vi "computeSetpoints.vi"(8 "idealSPFraction":dbl=0.7 format="%#_13g", 9 "Mdot":dbl, 10 "OffIdeal":dbl, 11 "MFCsIn":T1[](array[typedef]) {"mDot" format="%_4g"; "Setpoint" format="%.2g"; "MFCcapability"."MaxMdot" format="%_4g"; "MFCcapability"."MinMdot" format="%_4g"}) -> (1 "InactiveMFCs 2":T1[](array[typedef]) {"mDot" format="%_4g"; "Setpoint" format="%.2g"; "MFCcapability"."MaxMdot" format="%_4g"; "MFCcapability"."MinMdot" format="%_4g"}, 3 "ActiveMFCs":T1[](array[typedef]) {"mDot" format="%_4g"; "Setpoint" format="%.2g"; "MFCcapability"."MaxMdot" format="%_4g"; "MFCcapability"."MinMdot" format="%_4g"})   [LabVIEW 2021]
uses:
  MFCdescription.ctl
  MFCcapability.ctl
panel:
  out "mDotTotal":dbl
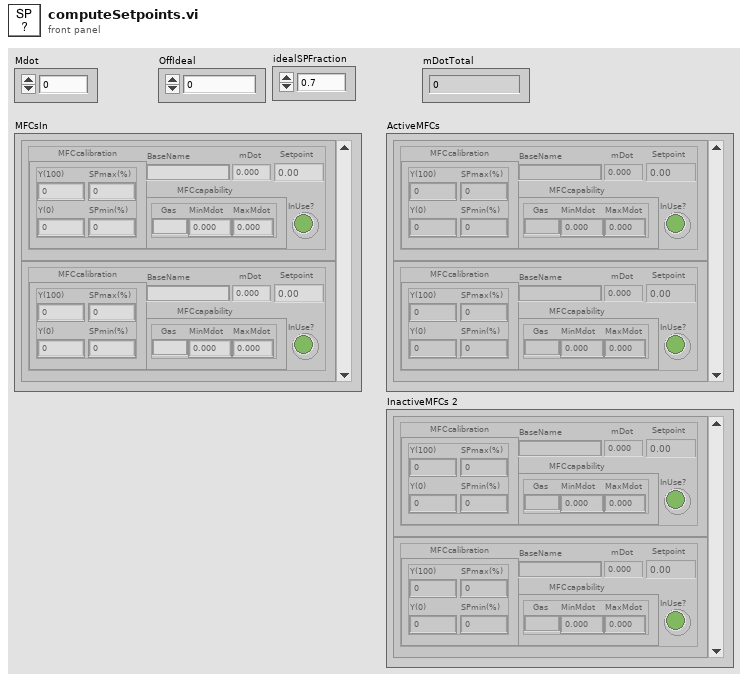
[diagram p1: front panel]
types:
  T1 = typedef "MFCdescription.ctl" = cluster{"BaseName":string, "MFCcalibration":cluster{"Y(100)":dbl, "Y(0)":dbl, "SPmin(%)":dbl, "SPmax(%)":dbl}, "MFCcapability":T2, "InUse?":bool, "Setpoint":dbl, "mDot":dbl}
  T2 = typedef "MFCcapability.ctl" = cluster{"Gas":string, "MinMdot":dbl, "MaxMdot":dbl}
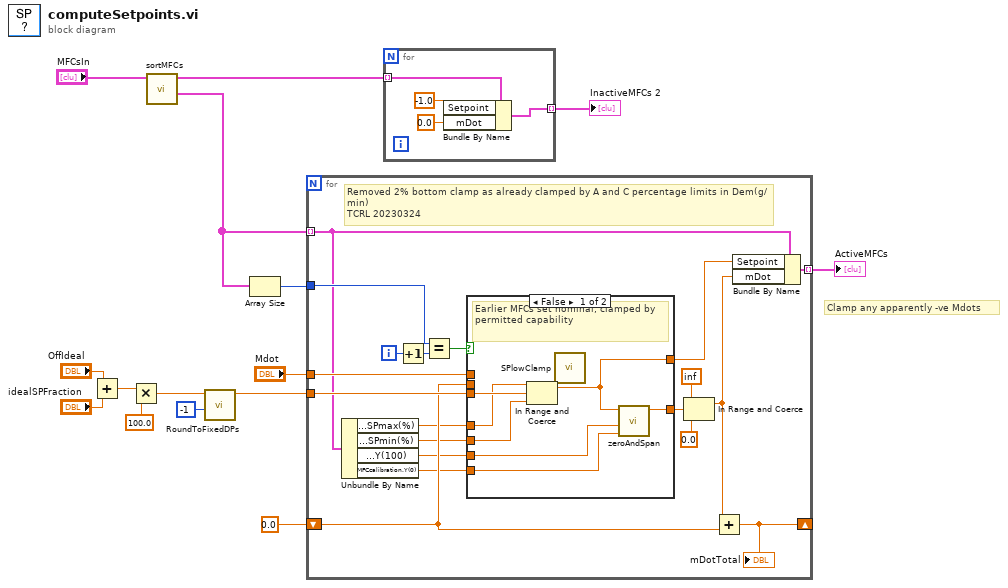
[diagram p0: block diagram]
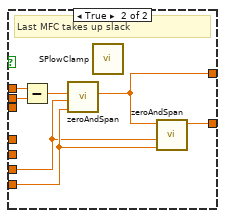
[diagram p2: hidden frame]
diagram:
  # "Clamp any apparently -ve Mdots"
  n1 = Add(x="OffIdeal", y="idealSPFraction") -> (x+y=w6:dbl)
  n2 = Multiply(x=w6, y=100.0) -> (x*y=w3:dbl)
  n3 = call "sortMFCs.vi"("MFCs"="MFCsIn") -> ("InUseMFCsascending"=w11:T1[], "notInUseMFCsascending"=w8:T1[])  [unwired: 7 in, 2 out]
  n4 = call "RoundToFixedDPs.vi"("Power of ten"=-1, "Number to round"=w3) -> ("Rounded number"=w5:dbl)  [unwired: 8 in, 1 out]
  n5 = Array Size(array=w11) -> (size(s)=w10:i32)
  n6 = for {
    tunnel: w5 -> [w33]
    tunnel: "Mdot" -> [w32]
    shift-right: [w28] -> _
    shift-left: 0.0 -> [w31]
    tunnel: w11 -> [w18] mode=indexing
    tunnel: w10 -> [w26]
    tunnel: [w22] -> w9 mode=indexing
    i -> [w27]
    # "Removed 2% bottom clamp as already clamped by A and C percentage limits in Dem(g/min)\nTCRL 20230324"
    n7 = Unbundle By Name(w18) -> ("MFCcalibration.SPmax(%)"=w17:dbl, "MFCcalibration.SPmin(%)"=w16:dbl, "MFCcalibration.Y(100)"=w30:dbl, "MFCcalibration.Y(0)"=w29:dbl)
    n8 = Increment(x=w27) -> (x+1=w25:i32)
    n9 = Equal?(x=w26, y=w25) -> (x = y?=w24:bool)
    n10 = case shown="False" w24 {
      tunnel: w33 -> [w37 _]
      tunnel: [w41 w43] -> w34
      tunnel: w32 -> [_ w48]
      tunnel: w31 -> [_ w47]
      tunnel: w30 -> [w40 w44]
      tunnel: w29 -> [w39 w45]
      tunnel: [w38 w42] -> w23
      tunnel: w17 -> [w36 _]
      tunnel: w16 -> [w35 _]
      frame False {
        # "Earlier MFCs set nominal, clamped by permitted capability"
        n11 = In Range and Coerce(upper limit=w36, x=w37, lower limit=w35) -> (coerced(x)=w38:dbl)  [unwired: 1 out]
        n12 = call "SPlowClamp.vi"() -> ()  [unwired: 15 in, 1 out]
        n13 = call "zeroAndSpan.vi"("Ymin"=w39, "Ymax"=w40, "MeasuredX"=w38) -> ("calibratedY"=w41:dbl)  [unwired: 6 in, 2 out]
      }
      frame True {
        # "Last MFC takes up slack"
        n14 = Subtract(x=w48, y=w47) -> (x-y=w46:dbl)
        n15 = call "zeroAndSpan.vi"("Ymin"=w45, "Ymax"=w44, "DesiredY"=w46) -> ("XToSet"=w42:dbl)  [unwired: 6 in, 2 out]
        n16 = call "SPlowClamp.vi"() -> ()  [unwired: 15 in, 1 out]
        n17 = call "zeroAndSpan.vi"("Ymin"=w45, "Ymax"=w44, "MeasuredX"=w42) -> ("calibratedY"=w43:dbl)  [unwired: 6 in, 2 out]
      }
    }
    n18 = In Range and Coerce(upper limit=inf, x=w34, lower limit=0.0) -> (coerced(x)=w19:dbl)  [unwired: 1 out]
    n19 = Add(x=w19, y=w31) -> (x+y=w28:dbl)
    "mDotTotal" <- w28
    n20 = Bundle By Name(cluster=w18, "Setpoint"=w23, "mDot"=w19) -> (w22:T1)
  }
  "ActiveMFCs" <- w9
  n21 = for {
    tunnel: w8 -> [w52] mode=indexing
    tunnel: [w50] -> w7 mode=indexing
    n22 = Bundle By Name(cluster=w52, "Setpoint"=-1.0, "mDot"=0.0) -> (w50:T1)
  }
  "InactiveMFCs 2" <- w7
